vi "Write Std Out with Redirection.vi"(0 "text":string) -> ()   [LabVIEW 2015]
uses:
  kernel32.dll
panel:
  out "error out":errorcluster
  in  "write .net":bool
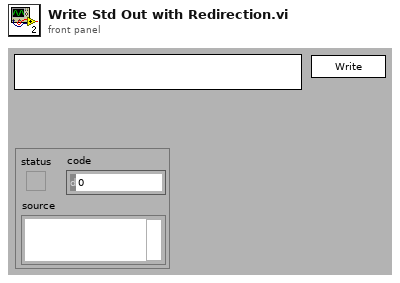
[diagram p1: front panel]
types:
  T1 = enum32{"invalid app kind", "Development System", "Run Time System", "Student Edition", "Embedded LabVIEW", "Evaluation", "Custom"}
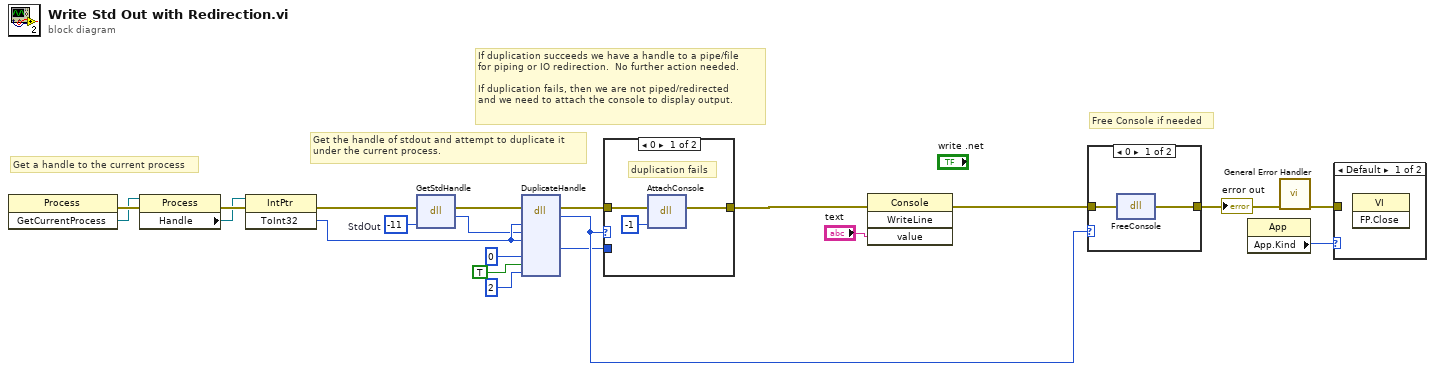
[diagram p0: block diagram]
diagram:
  w12 = -11  # StdOut
  # "If duplication succeeds we have a handle to a pipe/file\nfor piping or IO redirection.  No further action needed.\n\nIf duplication fails, then we are not piped/redirected\nand we need to attach the console to display output."
  # "Free Console if needed"
  # "Get the handle of stdout and attempt to duplicate it\nunder the current process."
  # "Get a handle to the current process"
  n1 = invoke class="Process" method="GetCurrentProcess"() -> (error out=w19:errorcluster, "GetCurrentProcess"=w10:refnum<k24>)  [unwired: 3 in, 1 out]
  n2 = property class="Process"(reference=w10, error in=w19) -> (error out=w18:errorcluster, "Handle"=w9:refnum<k24>)  [unwired: 1 out]
  n3 = invoke class="IntPtr" method="ToInt32"(reference=w9, error in=w18) -> (error out=w13:errorcluster, "ToInt32"=w20:i32)  [unwired: 1 in, 1 out]
  n4 = dll-call lib="kernel32.dll" fn="GetStdHandle"(error in=w13, "nStdHandle"=w12) -> (error out=w8:errorcluster, "return type"=w11:i32)  [unwired: 3 in, 1 out]
  n5 = dll-call lib="kernel32.dll" fn="DuplicateHandle"(error in=w8, "hSourceProcess"=w20, "hSourceHandle"=w11, "hTargetProcess"=w20, "dwDesirecAccess"=u16 0, "bInheritHandle"=TRUE, "dwOptions"=u16 2) -> (error out=w17:errorcluster, "return type"=w6:u8, "lpTargetHandle"=w4:i32)  [unwired: 9 in, 1 out]
  n6 = case shown="0" w6 {
    tunnel: w17 -> [w24 w25]
    tunnel: [w23 w25] -> w7
    tunnel: w4 -> [_ _]
    frame 0 {
      # "duplication fails"
      n7 = dll-call lib="kernel32.dll" fn="AttachConsole"(error in=w24, "arg1"=-1) -> (error out=w23:errorcluster)  [unwired: 4 in, 1 out]
    }
    frame Default {
      # "duplication succeeds"
    }
  }
  n8 = invoke class="Console" method="WriteLine"(error in=w7, "value"="text") -> (error out=w21:errorcluster)  [unwired: 2 in, 3 out]
  n9 = case shown="0" w6 {
    tunnel: w21 -> [w27 w28]
    tunnel: [w26 w28] -> w3
    frame 0 {
      n10 = dll-call lib="kernel32.dll" fn="FreeConsole"(error in=w27) -> (error out=w26:errorcluster)  [unwired: 2 in, 2 out]
    }
    frame Default {
    }
  }
  "error out" <- w3
  n11 = property class="App"() -> ("App.Kind"=w5:T1)  [unwired: 2 in, 2 out]
  n12 = call <vilib>:"General Error Handler.vi"("error in (no error)"=w3) -> ("error out"=w2:errorcluster)  [unwired: 10 in, 4 out]
  n13 = case shown="Default" w5 {
    tunnel: w2 -> [_ _]
    frame Default {
      n14 = invoke class="VI" method="FP.Close"() -> ()  [unwired: 3 in, 3 out]
    }
    frame "Development System" {
    }
  }
